vi "On Timeout Action Camera Setup.vi"(6 "Time":u32, 8 "error in (no error)":errorcluster, 11 "App in":refnum<class "App.lvclass">) -> (0 "error out":errorcluster, 3 "App out":refnum<class "App.lvclass">)   [LabVIEW 2020, in "AR Example.lvlib" / "App.lvclass"]
uses:
  App.lvclass
  App.lvclass/App.ctl
  UI/UI.lvclass
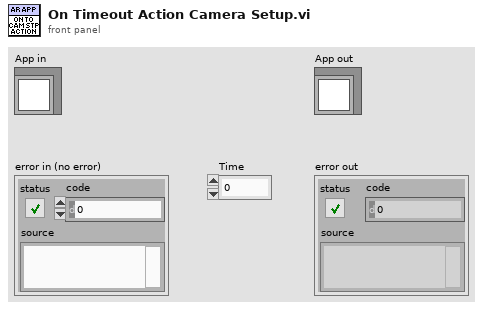
[diagram p1: front panel]
types:
  T1 = typedef "g_ar_toolkit.image.lvlib/Image Draw Offset.ctl" = cluster{"Left":i16, "Top":i16}
  T2 = typedef "g_ar_toolkit.image.lvlib/ARGB Image.ctl" = refnum<data-value>
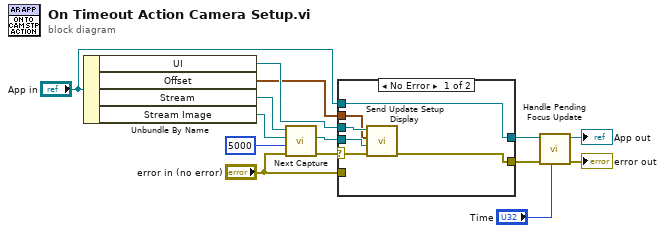
[diagram p0: block diagram]
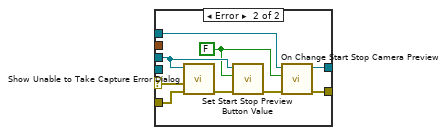
[diagram p2: hidden frame]
diagram:
  n1 = Unbundle By Name("App in") -> ("UI"=w12:refnum<class "UI.lvclass">, "Offset"=w6:T1, "Stream"=w1:refnum<class "Stream.lvclass">, "Stream Image"=w2:refnum<data-value>)
  n2 = call "Next Capture.vi"("error in (no error)"="error in (no error)", "timeout (Default: 1000 ms)"=u16 5000 ("timeout (ms)"), "ARGB Image Destination"=w2, "Stream in"=w1) -> ("error out"=w7:errorcluster, "ARGB Image (duplicate)"=w4:T2)  [unwired: 5 in, 1 out]
  n3 = case shown="No Error" w7 {
    selector: w7 -> [w19 w26]
    tunnel: w12 -> [w20 w22]
    tunnel: [w18 w27] -> w8
    tunnel: w4 -> [w17 _]
    tunnel: "error in (no error)" -> [_ w25]
    tunnel: w6 -> [w16 _]
    tunnel: [w15 w28] -> w10
    tunnel: "App in" -> [w15 w29]
    frame No Error {
      n4 = call-dynamic "Send Update Setup Display.vi"("error in (no error)"=w19, "Image"=w17, "Draw Offset"=w16, "UI in"=w20) -> ("error out"=w18:errorcluster)  [unwired: 7 in]
    }
    frame Error {
      w21 = FALSE ("Value")
      n5 = call-dynamic "Show Unable to Take Capture Error Dialog.vi"("error in (no error)"=w25, "Stream Start Error"=w26, "UI in"=w22) -> ("error out"=w24:errorcluster)  [unwired: 8 in]
      n6 = call-dynamic "Set Start Stop Preview Button Value.vi"("error in (no error)"=w24, "Values"=w21, "UI in"=w22) -> ("error out"=w23:errorcluster)  [unwired: 8 in]
      n7 = call "On Change Start Stop Camera Preview.vi"("error in (no error)"=w23, "Value"=w21, "App in"=w29) -> ("error out"=w27:errorcluster, "App out"=w28:refnum<class "App.lvclass">)  [unwired: 7 in]
    }
  }
  n8 = call "Handle Pending Focus Update.vi"("Time"="Time", "error in (no error)"=w8, "App in"=w10) -> ("error out"=→"error out":errorcluster, "App out"=→"App out":refnum<class "App.lvclass">)  [unwired: 7 in]
